vi "Exercise4_week2.vi"() -> ()   [LabVIEW 2015]
panel:
  out "ncr":dbl
  out "npr":dbl
  in  "r":dbl
  in  "n":dbl
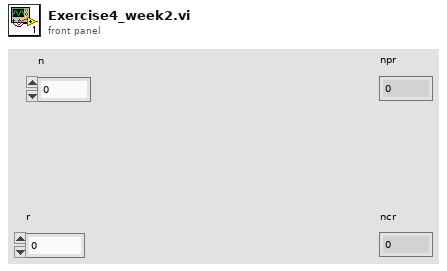
[diagram p1: front panel]
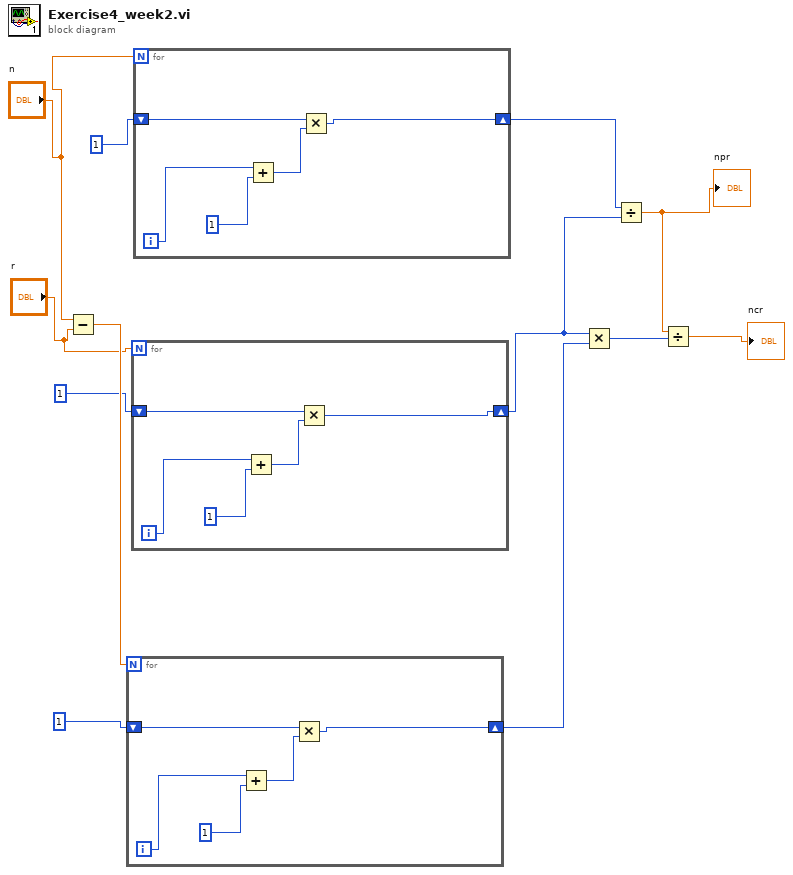
[diagram p0: block diagram]
diagram:
  n1 = Subtract(x="n", y="r") -> (x-y=w7:dbl)
  n2 = for {
    N: w7 -> [_]
    shift-right: [w13] -> w10
    shift-left: 1 -> [w14]
    i -> [w16]
    n3 = Add(x=w16, y=1) -> (x+y=w15:i32)
    n4 = Multiply(x=w14, y=w15) -> (x*y=w13:i32)
  }
  n5 = for {
    N: "r" -> [_]
    shift-right: [w19] -> w1
    shift-left: 1 -> [w18]
    i -> [w21]
    n6 = Add(x=w21, y=1) -> (x+y=w20:i32)
    n7 = Multiply(x=w18, y=w20) -> (x*y=w19:i32)
  }
  n8 = for {
    N: "n" -> [_]
    shift-right: [w23] -> w9
    shift-left: 1 -> [w24]
    i -> [w26]
    n9 = Add(x=w26, y=1) -> (x+y=w25:i32)
    n10 = Multiply(x=w24, y=w25) -> (x*y=w23:i32)
  }
  n11 = Multiply(x=w1, y=w10) -> (x*y=w12:i32)
  n12 = Divide(x=w9, y=w1) -> (x/y=w8:dbl)
  "npr" <- w8
  n13 = Divide(x=w8, y=w12) -> (x/y=→"ncr":dbl)
